vi "AlliGator Highlight Image ROI in Phasor Plot.vi"(0 "Source Image in":T1, 1 "Image Sum":T1, 2 "Source Image ROI Mask":T1, 5 "Phasor Plot Image in":T1, 7 "ROI":T2, 9 "[Corrected] Complex Phasor Array":csg[][](array[numeric]), 11 "Error In":errorcluster, 12 "Overlay Color":u32(colorbox)) -> (4 "Source Image out":T1, 6 "Phasor Plot Image out":T1, 10 "CPU (s)":dbl, 15 "Error Out":errorcluster)   [LabVIEW 2021, in "AlliGator Phasor Plot.lvlib"]
doc: "Highlights the phasors in the Phasor Plot image that corrspond to pixels in the Source Image ROI."
uses:
  AlliGator Phasor Plot.lvlib
  <vilib>/vision/Image Controls.llb/IMAQ Image.ctl
  Palette/Image Palette Information.ctl
  Image/Image Display Palette Type.ctl
  AlliGator Variables List.ctl
  AlliGator Settings List.ctl
  AlliGator Phasor Plot Reference Points.ctl
  40af3798-00bb-4b94-b92d-50ae21bc0bc0.vi
  Image/Global Rectangle Origin & Size.vi
  Variant/Variant to Data/Variant to Boolean.vi
  Variant/Variant to Data/Variant to I32.vi
  AlliGator Globals, Variables & Constants.lvlib
  AlliGator Phasor Ratio.lvlib
  Image/Image.lvlib
  AlliGator Source Image.lvlib
  <vilib>/vision/NI_Vision_Development_Module.lvlib
  Error/Error.lvlib
  Time/Time.lvlib
  Utilities/Utilities.lvlib
  AlliGator ROIs.lvlib
  AlliGator Settings.lvlib
  Variant/Variant to Data/Variant to Data.lvlib
  Palette/Palette.lvlib
panel:
  # "see the AlliGator License on the block diagram (Ctrl+E or Window:Show Block Diagram)"
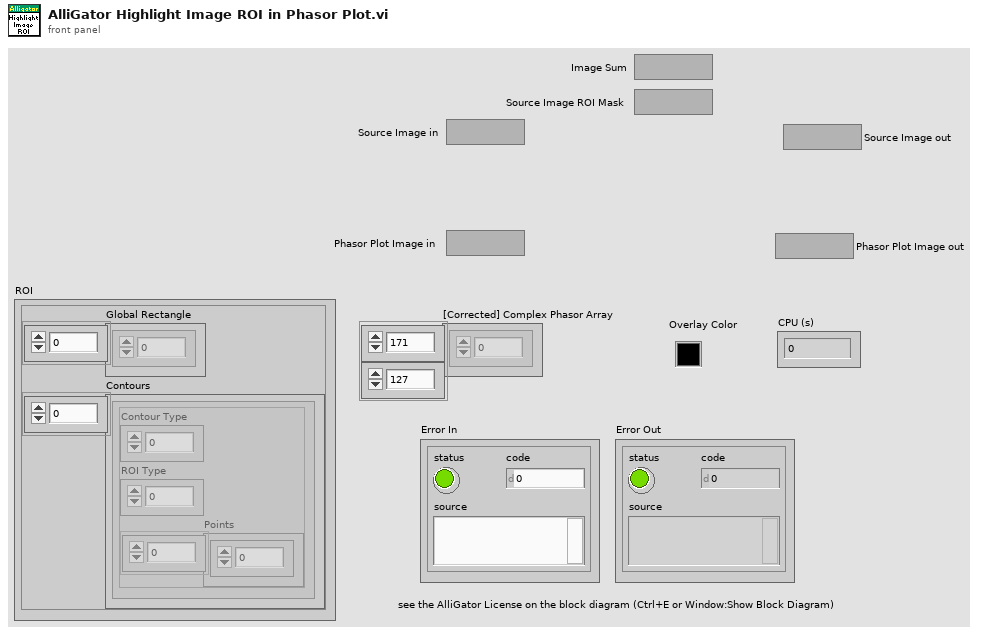
[diagram p1: front panel]
types:
  T1 = typedef "IMAQ Image.ctl" = refnum<image>
  T2 = cluster{"Global Rectangle":i32[], "Contours":cluster{"Contour Type":u32, "ROI Type":u32, "Points":i32[]}[]}
  T3 = typedef "Palette.lvlib/Image Palette Information.ctl" = cluster{"Palette Name [# Colors,int?,inv?]":string, "Palette Type":T4, "Palette Colors":u32[], "Interpolate?":bool}
  T4 = typedef "Image.lvlib/Image Display Palette Type.ctl" = u32
  T5 = typedef "AlliGator Globals, Variables & Constants.lvlib/AlliGator Variables List.ctl" = enum16{"---- GUI ----", "Initialization Status", "State Indicators Refnum", "Original AlliGator Menu Items", "Current Action Loop State", "Script in progress", "Playback", "Loop Playback", "Search ROI Used", "Search ROI", "Decay Graph Max Legend Size", "Intensity Graph Max Legend Size", "Decay Statistics Graph Max Legend Size", "Phasor Graph Max Legend Size", "Phasor Ratio Graph Max Legend Size", "Lifetime Graph Max Legend Size", "---- Files ----", "Export Dataset Frames as Individual Files", "Show Batch Export Help Balloons", "Frames in Dataset", "ptu File Frame Start Indices", "Current Frame in Dataset", "Current Frame Timestamp", "------ Python Plugins ------", "Python Plugins Information", "Python Session", "Valid Python Session?", "---- Source Image ----", "Dataset Loaded", "Dataset Metadata", "Dataset Channel", "Dataset Data Description", "Background Dataset Metadata", "Background Dataset Channel", "Background Dataset Data Description", "Background File Subtraction", "Background File Path", "Background File Pile-up Correction", "Background File Pixel Well Capacity", "Background File Scaling Factor", "Source Image ROIs", "Current Source Image ROI", "Source Image ROI Event Refnum", "X_Source Image Display Range", "X_Source Image Palette Information", "Source Image Palette List", "Source Image Scale", "Current Dataset Load Settings", "Source Image:ROI Overlay Color", "---- Image Profile Window ----", "Image Profile:Overlay ROI in Source Image", "Image Profile Window Event Refnum", "Image Profile:IntensityType", "Image Profile:Intensity Average Type", "Image Profile:Intensity-weighted SDV", "Image Profile:Box Profile Type", "Image Profile Window Open", "Image Profile:Plotted Fit Parameter", "X_Type of Displayed Image", "X_Time Gate Slider", "Dataset Path", "Source Image Overlay to Erase", "Is Displayed Image Accumulated", "White Light Image Modified", "Mask Image Modified", "Macrotime Gate Separation", "------ Phasor Graph -------", "Phasor Graph:Show Line", "---- Phasor Plot ---", "Phasor Plot Parameters Changed", "FLI Dataset Modified since last Phasor Plot Calculation", "Phasor Harmonics Data", "Selected Phasor Harmonics", "Phasor Harmonic Manager Event Refnum", "Phasor Plot ROIs", "Current Phasor Plot ROI", "Phasor Plot ROI Event Refnum", "Phasor Plot Image Reference Points", "Phasor Plot Computed", "Phasor Plot Palette Information", "Phasor Plot Palette List", "Phasor Ratio Palette Information", "Phasor Ratio Palette List", "Phasor Image Scale", "Phasor Plot Image Overlay to Erase", "Phasor Plot Image Elements to Update", "Current Phasor Plot Calculation Parameters", "Current Phasor Calibration Options", "Reset Cumulated Phasor Plot", "Phasor Ratio Reference 1", "Phasor Ratio Lifetime Reference 1", "Phasor Ratio Reference 1 Frequency", "Phasor Ratio Reference 2", "Phasor Ratio Lifetime Reference 2", "Phasor Ratio Reference 2 Frequency", "---- Decay Analysis ----", "Number of Selected Decays to Fit", "LS Fit Results", "LAR Fit Results", "BS Fit Results", "Last Decay Max - Min", "Best Fit Parameters", "Best Fit Parameter Names", "Actual Size X", "Actual Size Y", "Binning X", "Binning Y", "Actual # Gates", "Dataset Number", "Gates to...", "Gates Skipped", "Gates to keep", "Gate Step", "Gate Separation", "Reversed Gates", "Pile-up Correction", "Pixel Well Capacity", "Background Subtracted", "Background Subtraction Method", "Background Definition Range", "Background File (deprecated)", "Number of Dataset Accumulated", "Array of Accumulated Dataset Paths", "Do Averaged Datasets", "Destination File Path", "Process Plot Target", "Use 1/D as Phasor Frequency", "---- Decay Fit Parameter Map -----", "Decay Fit Parameter Map Palette Information", "Decay Fit Parameter Map Palette List", "Local Decay Graph Window Event Refnum", "------- Local Decay Window ---------", "Use normalized IRF for convolution", "----- Miscellaneous ----", "Skippable Dialog Windows Status"}
  T6 = typedef "AlliGator Settings.lvlib/AlliGator Settings List.ctl" = enum16{"GUI:Visible Settings Tab", "GUI:Last Run Version", "Source Image:Use Image Histogram for Contrast", "Source Image:Low Count Pixels Rejection Options", "Source Image:High Count Pixels Rejection Options", "Source Image:Use Image Brightness", "Source Image:Blend Overlay with Image Background", "Source Image:Use Fixed ROI Diameter", "Source Image:ROI Diameter", "Source Image:ROI Center Color", "Source Image:Peak Threshold", "Source Image:Intensity Threshold", "Source Image:Image Binning Options", "Source Image:Image Smoothing Options", "Source Image:Image Histogram Active", "Source Image:Invert Binary Mask", "Source Image:Hot Pixel Removal", "Source Image:Overlay Analyzed ROI Center", "Source Image:Auto-Adjust Contrast", "Source Image:Histogram Lower Percentile", "Source Image:Histogram Upper Percentile", "Source Image:Save Source Image", "Source Image:Scale Bar Options", "Source Image:Image Resolution (Pixel Size)", "Source Image:Flatfield Correction", "Data Information:Gate Width", "Data Information:Nanotime Gate Separation", "Data Information:Macrotime Gate Separation", "Data Information:Gate Step", "Data Information:# Gates", "Data Information:Gate Image Exposure", "Data Information:Gate Image Integration", "Data Information:Gates to Skip", "Data Information:Gates to Keep", "Data Information:Define Gates to", "Data Information:Channel Name", "Data Information:Available Channel Names", "Data Information:Channel Arithmetic", "Data Information:Background File Subtraction", "Data Information:Background File", "Data Information:Background Scaling Factor", "Data Information:Background Pile-up Correction", "Data Information:Background Pixel Well Capacity", "Data Information:Laser Period", "Data Information:SYNC Period", "Data Information:Pile-up Correction", "Data Information:Pixel Well Capacity", "Data Information:Dataset Scaling Factor", "Fluorescence Decay_Decay Pre-Processing:Reverse Gates", "Fluorescence Decay_Decay Pre-Processing:Verbose Decay Pre-Processing", "Fluorescence Decay_Decay Pre-Processing:Use Decay Pre-Processing", "Fluorescence Decay_Decay Pre-Processing:Background Subtraction", "Fluorescence Decay_Decay Pre-Processing:Background Definition Range", "Fluorescence Decay_Decay Pre-Processing:Baseline Subtraction Method", "Fluorescence Decay_Decay Pre-Processing:Operations Order", "Fluorescence Decay_Decay Pre-Processing:Smoothing Parameter", "Fluorescence Decay_Decay Pre-Processing:Shift Decay", "Fluorescence Decay_Decay Pre-Processing:Decay Shift Parameters", "Fluorescence Decay_Decay Pre-Processing:Fold Decay", "Fluorescence Decay_Decay Pre-Processing:# Folds", "Fluorescence Decay_Decay Pre-Processing:1-Normalize Decay", "Fluorescence Decay_Decay Pre-Processing:[0-1]-Normalize Decay", "Fluorescence Decay_Decay Pre-Processing:Smoothen Decay", "Fluorescence Decay_Decay Pre-Processing:Extrapolate Decay", "Fluorescence Decay_Decay Pre-Processing:Use Periodicity", "Fluorescence Decay_Decay Pre-Processing:Use Cursors", "Fluorescence Decay_Decay Pre-Processing:Tail Fraction", "Fluorescence Decay_Decay Pre-Processing:Head Fraction", "Fluorescence Decay_Decay Pre-Processing:Additional Points", "Fluorescence Decay_Decay Pre-Processing:Straighten Decay", "Fluorescence Decay_Decay Pre-Processing:Constant Background", "Fluorescence Decay_Decay Pre-Processing:Pixel-Normalize Decay", "Fluorescence Decay_Advanced Analysis:Extract IRF instead of Decay", "Fluorescence Decay_Advanced Analysis:IRF Extraction Options", "Fluorescence Decay_Advanced Analysis:IRF Optimization Options", "Fluorescence Decay_Advanced Analysis:Square Pulse Options", "Fluorescence Decay_Advanced Analysis:IRF Order", "Fluorescence Decay_Advanced Analysis:IRF Time Constants", "Fluorescence Decay_Advanced Analysis:Wavelet Analysis Options", "Fluorescence Decay_Advanced Analysis:Average Lifetime Options", "Fluorescence Decay_Fit Options:Fit Options", "Fluorescence Decay_Fit Options:Use Legacy Fitting Approach", "Fluorescence Decay_Fit Options:Use Data Information Laser Period", "Fluorescence Decay_Fit Parameters:Displayed Fit Parameters", "Fluorescence Decay_Fit Parameters:Fit Parameter Constraints", "Fluorescence Decay_Fit Parameters:Export Tabulated Results", "Fluorescence Decay_Fit Parameters:MLE Baseline Offset Type", "Fluorescence Decay_Fit Parameters:MLE Baseline Offset", "Fluorescence Decay_Fit Parameters:Guess Parameter Names", "Fluorescence Decay_Fit Parameters:Guess Parameter Values", "Fluorescence Decay_Fit Parameters:Guess Parameters Options", "Fluorescence Decay_Styles:Show Last Decay Only", "Fluorescence Decay_Styles:Decay Graph Color Array", "Fluorescence Decay:Decay Graph Active", "Fluorescence Decay Statistics:Min Peak Value", "Fluorescence Decay Statistics:Reject Low Decay Peak Pixels", "Fluorescence Decay Statistics:Reject High Decay Peak Pixels", "Fluorescence Decay Statistics:Max Peak Value", "Time Traces:Use File Timestamp", "Time Traces:Time Step", "Time Traces:Use Intensity Correction File", "Time Traces:Intensity Correction File", "Phasor Plot:Phasor Plot Smoothing Options", "Phasor Plot:Phasor Plot Size", "Phasor Plot:Phasor Plot Graphics Options", "Phasor Plot:Cumulative Phasor Plot", "Phasor Plot:Use Phasor Brightness", "Phasor Plot:Blend Overlay with Phasor Background", "Phasor Plot:Save Phasor Plot", "Phasor Plot:Show References", "Phasor Plot:Phasor Ratio Decay Range", "Phasor Plot:Exponential Fading", "Phasor Plot:Phasor Ratio Reference Colors", "Phasor Plot:Reference Radius", "Phasor Plot:Show Color Map Vertices", "Phasor Plot:Phasor Plot Active", "Phasor Plot:Phasor Ratio Color Map Type", "Phasor Plot:Phasor Ratio Color Map", "Phasor Plot:Phasor Ratio Display Range", "Phasor Plot:Selected Image ROI(s)", "Phasor Plot:All Image ROIs", "Phasor Plot:Selected Phasor Plot ROI(s)", "Phasor Plot:All Phasor Plot ROIs", "Phasor Plot:Phasor Ratio Color-Coded Quantity", "Phasor Plot:Store Phasor Harmonics", "Phasor Plot:Draw Reference Segment", "Phasor Plot:User-Defined Quantity", "Phasor Graph:Phasor Frequency", "Phasor Graph:Phasor Ratio Type", "Phasor Graph:Pixel-level Phasor Computation", "Phasor Graph:Save Phasor Graph", "Phasor Graph:Phasor Graph Active", "Phasor Graph:Phasor SDV Options", "Phasor Calibration:Use Backup Calibration if needed", "Phasor Graph:Define Shortest Lifetime as", "Phasor Calibration:Backup Calibration Type", "Phasor Calibration:Calibration Type", "Phasor Calibration:Calibration Lifetime", "Phasor Calibration:Calibration Map Algorithm", "Single-Exponential Phasor Locus (SEPL):Gate Parameters", "Single-Exponential Phasor Locus (SEPL):User-defined Gate", "Single-Exponential Phasor Locus (SEPL):User-defined IRF", "Single-Exponential Phasor Locus (SEPL):Phasor Parameters", "Single-Exponential Phasor Locus (SEPL):Decay & IRF Parameters", "Single-Exponential Phasor Locus (SEPL):Display Parameters", "Lifetime Analysis:Decay Analysis Parameters", "Lifetime Analysis:Lifetime Map Active", "Plugins:Python Settings", "Miscellaneous:Verbose Mode", "Miscellaneous:Beep after Script", "Miscellaneous:Saved Image File Format", "Miscellaneous:Exported Gate Image Settings", "Miscellaneous:Include Loading in Timing", "Miscellaneous:Verbose Settings Mode", "Miscellaneous:Histogram Options", "Miscellaneous:Beep on Error", "Miscellaneous:# Logical Processors Used", "Miscellaneous:ROI Description Max Characters", "Miscellaneous:Verbose Error Mode", "Miscellaneous:Transparent Mask Color"}
  T7 = typedef "AlliGator Phasor Ratio.lvlib/AlliGator Phasor Plot Reference Points.ctl" = cluster{"O_h":dbl, "O_v":dbl, "1_h":dbl, "1_v":dbl}
  T8 = typedef "ROI Descriptor" = cluster{"Global Rectangle":i32[], "Contours":cluster{"ID":enum32{"External", "Internal"}, "Type":u32, "Coordinates":i32[]}[]}
  T9 = cluster{"histogram":u32[], "Minimal Value":sgl, "Maximal Value":sgl, "Starting Value":sgl, "Interval Width":sgl, "Mean Value":sgl, "Standard  Variation":sgl, "Area (pixels)":i32}
  T10 = cluster{"Red (or Hue) value":u8, "Green (or Sat) value":u8, "Blue (or Light or Val) value":u8}
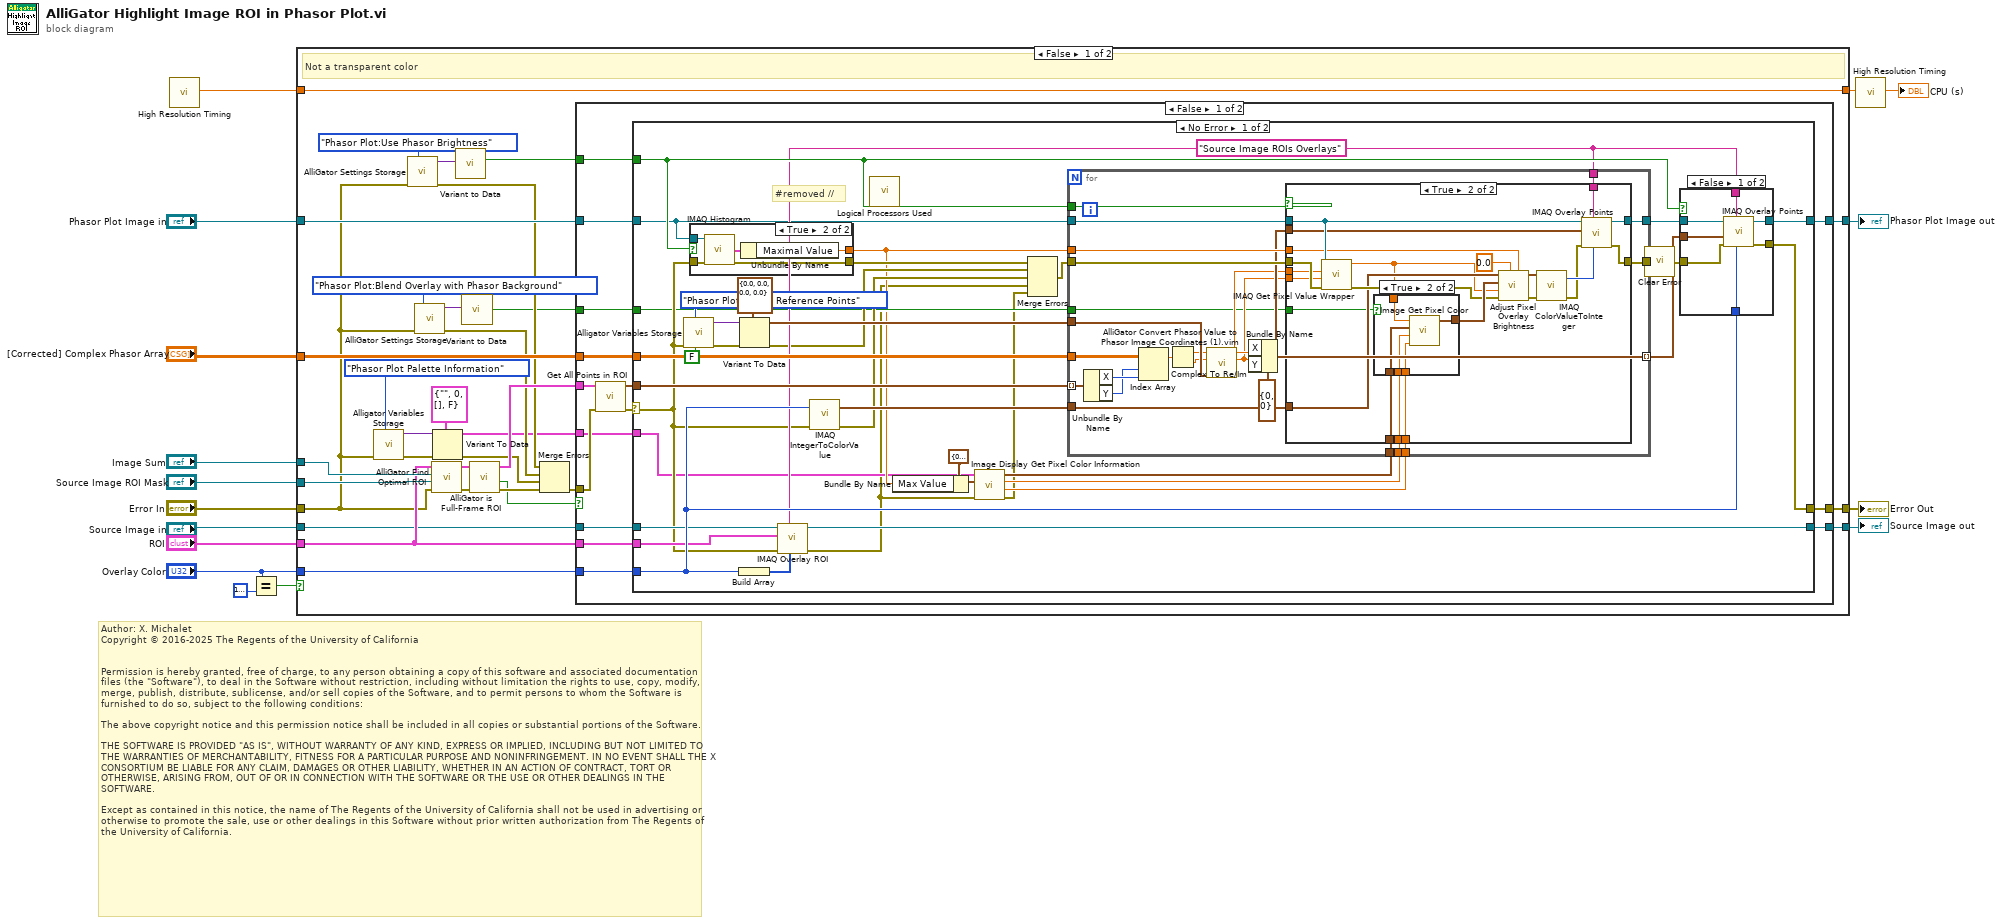
[diagram p0: block diagram]
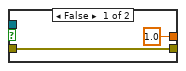
[diagram p2: hidden frame]
diagram:
  # "Author: X. Michalet\nCopyright © 2016-2025 The Regents of the University of California\n \n\nPermission is hereby granted, free of charge, to any person obtaining a copy of this software and associated documentation files (the \"Software\"), to deal in the Software without restriction, including without limitation the rights to use, copy, modify, merge, publish, distribute, sublicense, and/or sell copies of the Software, and to permit persons to whom the Software is furnished to do so, subject to the following conditions:\n\nThe above copyright notice and this permission notice shall be included in all copies or substantial portions of the Software.\n\nTHE SOFTWARE IS PROVIDED \"AS IS\", WITHOUT WARRANTY OF ANY KIND, EXPRESS OR IMPLIED, INCLUDING BUT NOT LIMITED TO THE WARRANTIES OF MERCHANTABILITY, FITNESS FOR A PARTICULAR PURPOSE AND NONINFRINGEMENT. IN NO EVENT SHALL THE X CONSORTIUM BE LIABLE FOR ANY CLAIM, DAMAGES OR OTHER LIABILITY, WHETHER IN AN ACTION OF CONTRACT, TORT OR OTHERWISE, ARISING FROM, OUT OF OR IN CONNECTION WITH THE SOFTWARE OR THE USE OR OTHER DEALINGS IN THE SOFTWARE.\n\nExcept as contained in this notice, the name of The Regents of the University of California shall not be used in advertising or otherwise to promote the sale, use or other dealings in this Software without prior written authorization from The Regents of the University of California."
  n1 = call "High Resolution Timing.vi"() -> ("elapsed (relative) seconds"=w11:dbl)  [unwired: 17 in, 2 out]
  n2 = Equal?(x="Overlay Color", y=u32 16777216 ("Overlay Color")) -> (x = y?=w9:bool)
  n3 = case shown="False" w9 {
    tunnel: "[Corrected] Complex Phasor Array" -> [w48 _]
    tunnel: "Error In" -> [w20 w179]
    tunnel: [w36 w179] -> w14
    tunnel: "Image Sum" -> [w47 _]
    tunnel: "Overlay Color" -> [w46 _]
    tunnel: w11 -> [w45 w178]
    tunnel: [w45 w178] -> w10
    tunnel: "Source Image ROI Mask" -> [w44 _]
    tunnel: "Phasor Plot Image in" -> [w41 w177]
    tunnel: [w40 w177] -> w5
    tunnel: "ROI" -> [w39 _]
    tunnel: "Source Image in" -> [w38 w176]
    tunnel: [w37 w176] -> w2
    frame False {
      # "Not a transparent color"
      n4 = call "Alligator Variables Storage.vi"("AlliGator Variable"=AlliGator_Variables_List."Phasor Plot Palette Information" ("Alligator Variable"), "Error In"=w20) -> ("Error Out"=w19:errorcluster, "Data out"=w23:variant)  [unwired: 7 in, 1 out]
      n5 = call "AlliGator Settings Storage.vi"("AlliGator Settings List"=AlliGator_Settings_List."Phasor Plot:Use Phasor Brightness", "Error In"=w20) -> ("Error Out"=w29:errorcluster, "Variant Data out"=w32:variant)  [unwired: 8 in]
      n6 = call "AlliGator Settings Storage.vi"("AlliGator Settings List"=AlliGator_Settings_List."Phasor Plot:Blend Overlay with Phasor Background", "Error In"=w20) -> ("Error Out"=w25:errorcluster, "Variant Data out"=w26:variant)  [unwired: 8 in]
      n7 = call "AlliGator Find Optimal ROI.vi"("error in (no error)"=w20, "ROI Mask"=w44, "Image Sum"=w47, "ROI Descriptor in"=w39) -> ("error out"=w43:errorcluster, "ROI Descriptor out"=w42:T8)  [unwired: 5 in, 1 out]
      n8 = Variant To Data(error in=w19, type=T3 {"Palette Name [# Colors,int?,inv?]"="", "Palette Type"=0, "Palette Colors"=[], "Interpolate?"=FALSE} ("Image Display Palette Information"), Variant=w23) -> (data=w17:T3, error out=w18:errorcluster)
      n9 = call-poly "Variant to Data.vi"("Variant"=w32) -> ("Value"=w31:bool)  [unwired: 8 in]
      n10 = call-poly "Variant to Data.vi"("Variant"=w26) -> ("Value"=w24:bool)  [unwired: 8 in]
      n11 = call "AlliGator is Full-Frame ROI.vi"("error in (no error)"=w43, "ROI Descriptor in"=w42) -> ("error out"=w35:errorcluster, "Full-Frame ROI?"=w33:bool, "ROI Descriptor (dup)"=w34:T8)  [unwired: 7 in]
      n12 = Merge Errors(w29, w25, w18, w35) -> (w30:errorcluster)
      n13 = case shown="False" w33 {
        tunnel: w48 -> [w63 _]
        tunnel: w31 -> [w62 _]
        tunnel: w46 -> [w61 _]
        tunnel: w41 -> [w58 w173]
        tunnel: [w57 w173] -> w40
        tunnel: w39 -> [w56 _]
        tunnel: w38 -> [w55 w174]
        tunnel: [w54 w174] -> w37
        tunnel: [w53 w175] -> w36
        tunnel: w30 -> [w52 w175]
        tunnel: w34 -> [w51 _]
        tunnel: w24 -> [w50 _]
        tunnel: w17 -> [w49 _]
        frame False {
          n14 = call "Get All Points in ROI.vi"("Error In"=w52, "ROI Descriptor"=w51) -> ("Error Out"=w59:errorcluster, "Point Array"=w60:cluster{"X":i32, "Y":i32}[])  [unwired: 8 in]
          n15 = case shown="No Error" w59 {
            selector: w59 -> [w74 _]
            tunnel: w63 -> [w101 _]
            tunnel: w62 -> [w100 _]
            tunnel: w61 -> [w99 _]
            tunnel: w56 -> [w98 _]
            tunnel: w60 -> [w90 _]
            tunnel: w58 -> [w79 w171]
            tunnel: [w78 w171] -> w57
            tunnel: w55 -> [w77 w172]
            tunnel: [w76 w172] -> w54
            tunnel: [w75 _] -> w53
            tunnel: w50 -> [w73 _]
            tunnel: w49 -> [w69 _]
            frame No Error {
              w84 = "Source Image ROIs Overlays" ("Group")
              # "#removed //"
              n16 = call "Alligator Variables Storage.vi"("Get(F)/Set"=FALSE, "AlliGator Variable"=AlliGator_Variables_List."Phasor Plot Image Reference Points" ("Alligator Variable"), "Error In"=w74) -> ("Error Out"=w93:errorcluster, "Data out"=w95:variant)  [unwired: 6 in, 1 out]
              n17 = case shown="True" w100 {
                tunnel: w79 -> [_ w108]
                tunnel: [w102 w106] -> w87
                tunnel: [sgl 1.0 ("Maximal Value") w105] -> w70
                tunnel: w74 -> [w102 w104]
                frame False {
                }
                frame True {
                  n18 = call "IMAQ Histogram"("error in (no error)"=w104, "Image"=w108) -> ("error out"=w106:errorcluster, "Histogram Report"=w107:T9)  [unwired: 8 in]
                  n19 = Unbundle By Name(w107) -> ("Maximal Value"=w105:sgl)
                }
              }
              n20 = Build Array(w99) -> (w91:u32[])
              n21 = Variant To Data(error in=w93, type=T7 {"O_h"=0.0, "O_v"=0.0, "1_h"=0.0, "1_v"=0.0} ("Phasor Plot Reference Points"), Variant=w95) -> (data=w92:T7, error out=w81:errorcluster)
              n22 = call "IMAQ Overlay ROI"("Colors (Green)"=w91, "Group"=w84, "error in (no error)"=w74, "ROI Descriptor"=w98, "Image"=w77) -> ("error out"=w65:errorcluster, "Image Out"=w76:T1)  [unwired: 5 in]
              n23 = call "IMAQ IntegerToColorValue"("error in (no error)"=w74, "U32 value"=w99) -> ("error out"=w80:errorcluster, "Color Value"=w85:T10)  [unwired: 3 in, 2 out]
              n24 = call "Logical Processors Used.vi"() -> ()  [unwired: 6 in, 1 out]
              n25 = Bundle By Name(cluster=cluster{"Min Value":dbl, "Max Value":dbl} {"Min Value"=0.0, "Max Value"=nan} ("Image Display Range"), "Max Value"=w70) -> (w72:cluster{"Min Value":dbl, "Max Value":dbl})
              n26 = call "Image Display Get Pixel Color Information.vi"("Error In"=w65, "Image Display Range"=w72, "Image Display Palette Information"=w69) -> ("Error Out"=w64:errorcluster, "Image Scale Factor"=w66:dbl, "Image Range Min Value"=w67:dbl, "1D Color value array"=w68:cluster{"Red":u8, "Green":u8, "Blue":u8}[])  [unwired: 5 in]
              n27 = Merge Errors(w87, w81, w80, w65, w64) -> (w82:errorcluster)
              n28 = for {
                tunnel: w101 -> [w141]
                tunnel: w92 -> [w140]
                tunnel: w90 -> [w138] mode=indexing
                tunnel: [w128] -> w89 mode=indexing
                tunnel: w100 -> [w134]
                tunnel: w70 -> [w129]
                tunnel: w85 -> [w122]
                tunnel: w84 -> [w127]
                tunnel: w82 -> [w131]
                tunnel: [w130] -> w86
                tunnel: w79 -> [w133]
                tunnel: [w132] -> w88
                tunnel: w73 -> [w121]
                tunnel: w68 -> [w120]
                tunnel: w67 -> [w119]
                tunnel: w66 -> [w118]
                n29 = Unbundle By Name(w138) -> ("X"=w124:i32, "Y"=w123:i32)
                n30 = Index Array(array=w141, index (row)=w123, index (col)=w124) -> (element=w139:csg)
                n31 = Complex To Re/Im(x + iy=w139) -> (x=w137:sgl, y=w136:sgl)
                n32 = call "AlliGator Convert Phasor Value to Phasor Image Coordinates (1).vim"("Phasor Plot Reference Points"=w140, "Phasor s"=w136, "Phasor g"=w137) -> ("Phasor Plot y"=w125:dbl, "Phasor Plot x"=w126:dbl)  [unwired: 7 in]
                n33 = Bundle By Name(cluster=cluster{"X":i32, "Y":i32} {"X"=0, "Y"=0} ("Point"), "X"=w126, "Y"=w125) -> (w128:cluster{"X":i32, "Y":i32})
                n34 = case shown="True" w134 {
                  tunnel: w133 -> [w143 w163]
                  tunnel: [w143 w165] -> w132
                  tunnel: w131 -> [w142 w164]
                  tunnel: [w142 w159] -> w130
                  tunnel: w129 -> [_ w149]
                  tunnel: w128 -> [_ w162]
                  tunnel: w127 -> [_ w158]
                  tunnel: w126 -> [_ w157]
                  tunnel: w125 -> [_ w156]
                  tunnel: w122 -> [_ w153]
                  tunnel: w121 -> [_ w148]
                  tunnel: w120 -> [_ w147]
                  tunnel: w119 -> [_ w146]
                  tunnel: w118 -> [_ w145]
                  frame False {
                  }
                  frame True {
                    n35 = call "IMAQ Get Pixel Value Wrapper.vi"("Error In"=w164, "Y Coordinate"=w156, "X Coordinate"=w157, "Image"=w163) -> ("Error Out"=w154:errorcluster, "Pixel Value"=w144:sgl)  [unwired: 5 in, 1 out]
                    n36 = case shown="True" w148 {
                      tunnel: [_ w170] -> w155
                      tunnel: w147 -> [_ w169]
                      tunnel: w146 -> [_ w168]
                      tunnel: w145 -> [_ w167]
                      tunnel: w144 -> [_ w166]
                      frame False {
                      }
                      frame True {
                        n37 = call "Image Get Pixel Color.vi"("Image Scale Factor"=w167, "Image Range Min Value"=w168, "1D Color value array"=w169, "Image Pixel Value"=w166) -> ("Pixel Color Value (black)"=w170:T10)  [unwired: 7 in]
                      }
                    }
                    n38 = call "Adjust Pixel Overlay Brightness.vi"("Scale Max"=w149, "Scale Min"=0.0, "Error In"=w154, "Pixel in"=w144, "Pixel Color Value (black)"=w155, "Overlay Color Value in"=w153) -> ("Error Out"=w152:errorcluster, "Overlay Color Value out"=w151:T10)  [unwired: 4 in]
                    n39 = call "IMAQ ColorValueToInteger"("error in (no error)"=w152, "Color Value"=w151) -> ("error out"=w160:errorcluster, "U32 value"=w161:u32)  [unwired: 3 in, 2 out]
                    n40 = call "IMAQ Overlay Points"("Color"=w161, "Group"=w158, "error in (no error)"=w160, "Point"=w162, "Image"=w163) -> ("error out"=w159:errorcluster, "Image Out"=w165:T1)  [unwired: 5 in]
                  }
                }
              }
              n41 = call "Clear Error.vi"("Error In"=w86) -> ("no Error Out"=w83:errorcluster)  [unwired: 8 in]
              n42 = case shown="False" w100 {
                tunnel: w88 -> [w115 w117]
                tunnel: [w114 w117] -> w78
                tunnel: [w113 w116] -> w75
                tunnel: w84 -> [w112 _]
                tunnel: w99 -> [w111 _]
                tunnel: w89 -> [w110 _]
                tunnel: w83 -> [w109 w116]
                frame False {
                  n43 = call "IMAQ Overlay Points"("Color"=w111, "Group"=w112, "error in (no error)"=w109, "Array of Points"=w110, "Image"=w115) -> ("error out"=w113:errorcluster, "Image Out"=w114:T1)  [unwired: 5 in]
                }
                frame True {
                  # "this has been computed in the main For Loop"
                }
              }
            }
            frame Error {
              # "empty or no ROI"
            }
          }
        }
        frame True {
        }
      }
    }
    frame True {
    }
  }
  "Error Out" <- w14
  "Phasor Plot Image out" <- w5
  "Source Image out" <- w2
  n44 = call "High Resolution Timing.vi"("relative seconds (NaN)"=w10) -> ("elapsed (relative) seconds"=→"CPU (s)":dbl)  [unwired: 16 in, 2 out]
